vi "Set Icon.vi"(6 "Variant in":variant, 7 "Shift Pressed?":bool, 8 "error in (no error)":errorcluster, 10 "QD Combo Box Ref":refnum<vi>, 11 "QD Launch VI Ref":refnum<vi>) -> (0 "error out":errorcluster, 4 "Variant out":variant)   [LabVIEW 2017]
doc: "Replaces active VI Icon. New icon, by default, has a frame with black header and text with active VI name. Enter <b>-?</b> to display help window.\n\nDefault Shortcut - [N]"
uses:
  <vilib>/LabVIEW Icon API/API_User Layer Data.ctl
  <vilib>/Utility/miscctls.llb/LVPoint32TypeDef.ctl
  <vilib>/picture/picture.llb/imagedata.ctl
  <vilib>/LabVIEW Icon API/LabVIEW Icon API.lvlib
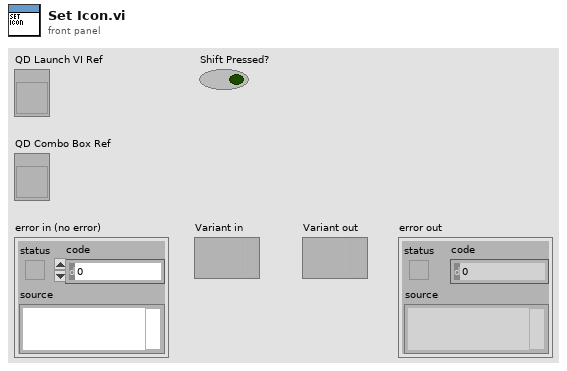
[diagram p1: front panel]
types:
  T1 = typedef "LabVIEW Icon API.lvlib/API_User Layer Data.ctl" = cluster{"Layer name":string, "Origin":T2, "Icon image data":T3}
  T2 = typedef "LVPoint32TypeDef.ctl" = cluster{"Horizontal":i32, "Vertical":i32}
  T3 = typedef "imagedata.ctl" = cluster{"image type":i32, "image depth":i32, "image":u8[], "mask":u8[], "colors":u32[], "Rectangle":cluster{"left":i16, "top":i16, "right":i16, "bottom":i16}}
  T4 = typedef "Settings.ctl" = cluster{"main text":string, "header text":string, "color":u32, "dark?":bool, "frame":T5, "format":T6, "number of lines":i32, "header?":bool, "shift":cluster{"x":i16, "y":i16}}
  T5 = typedef "Template Frame.ctl" = enum16{"none", "compact lib"}
  T6 = typedef "Text Format.ctl" = enum16{"none"}
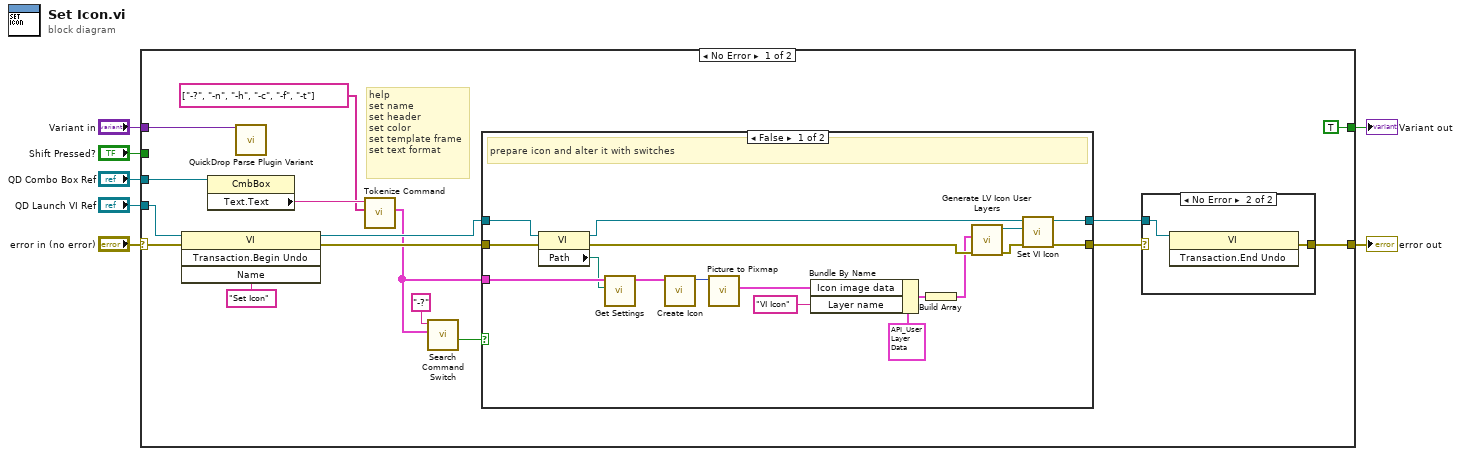
[diagram p0: block diagram]
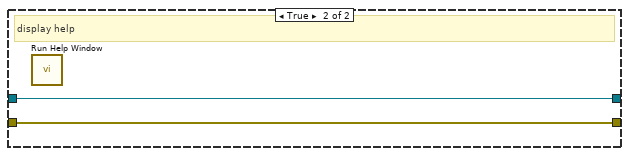
[diagram p2: hidden frame]
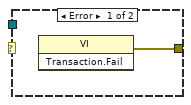
[diagram p3: hidden frame]
diagram:
  n1 = case shown="No Error" "error in (no error)" {
    selector: "error in (no error)" -> [w22 w46]
    tunnel: [w20 w46] -> w6
    tunnel: "QD Launch VI Ref" -> [w21 _]
    tunnel: "Shift Pressed?" -> [_ _]
    tunnel: "QD Combo Box Ref" -> [w18 _]
    tunnel: "Variant in" -> [w23 _]
    tunnel: [TRUE _] -> w1
    frame No Error {
      # "help\nset name\nset header\nset color\nset template frame\nset text format"
      n2 = invoke class="VI" method="Transaction.Begin Undo"(reference=w21, error in=w22, "Name"="Set Icon" ("Undo Name")) -> (reference out=w12:refnum<vi>, error out=w11:errorcluster)  [unwired: 1 in, 2 out]
      n3 = property class="CmbBox"(reference=w18) -> ("Text.Text"=w16:string)  [unwired: 1 in, 2 out]
      n4 = call <vilib>:"QuickDrop Parse Plugin Variant.vi"("QDKS Variant in"=w23) -> ()  [unwired: 12 in, 3 out]
      n5 = call "Tokenize Command.vi"("switches in"=string[] ["-?", "-n", "-h", "-c", "-f", "-t"], "command in"=w16) -> ("switches out"=w10:cluster{"switch":string, "argument":string}[])  [unwired: 7 in, 2 out]
      n6 = call "Search Command Switch.vi"("switches"=w10, "switch in"="-?" ("y")) -> ("found?"=w14:bool)  [unwired: 7 in, 2 out]
      n7 = case shown="False" w14 {
        tunnel: w10 -> [w39 _]
        tunnel: w12 -> [w38 w42]
        tunnel: w11 -> [w37 w41]
        tunnel: [w25 w42] -> w9
        tunnel: [w24 w41] -> w8
        frame False {
          # "prepare icon and alter it with switches"
          n8 = property class="VI"(reference=w38, error in=w37) -> (reference out=w29:refnum<vi>, error out=w40:errorcluster, "Path"=w36:path)
          n9 = call "Get Settings.vi"("VI path"=w36, "switches"=w39) -> ("settings"=w35:T4)  [unwired: 9 in]
          n10 = call "Create Icon.vi"("settings"=w35) -> ("new picture"=w30:picture)  [unwired: 10 in]
          n11 = call <vilib>:"Picture to Pixmap.vi"("picture"=w30) -> ("image data"=w26:T3)  [unwired: 9 in, 1 out]
          n12 = Bundle By Name(cluster=T1 {"Layer name"="", "Origin"={"Horizontal"=0, "Vertical"=0}, "Icon image data"={"image type"=0, "image depth"=0, "image"=[], "mask"=[], "colors"=[], "Rectangle"={"left"=0, "top"=0, "right"=0, "bottom"=0}}} ("User layer"), "Icon image data"=w26, "Layer name"="VI Icon") -> (w33:T1)
          n13 = Build Array(w33) -> (w32:T1[])
          n14 = call <vilib>:"Generate LV Icon User Layers.vi"("error in (no error)"=w40, "User layers"=w32) -> ("error out"=w27:errorcluster, "Icon out"=w28:refnum<class "Icon.lvclass">)  [unwired: 8 in]
          n15 = call <vilib>:"Set VI Icon.vi"("error in (no error)"=w27, "Icon"=w28, "VI Refnum in"=w29) -> ("error out"=w24:errorcluster, "VI Refnum out"=w25:refnum<vi>)  [unwired: 7 in]
        }
        frame True {
          # "display help"
          n16 = call "Run Help Window.vi"() -> ()  [unwired: 11 in, 1 out]
        }
      }
      n17 = case shown="No Error" w8 {
        tunnel: [w43 w45] -> w20
        tunnel: w9 -> [_ w44]
        frame Error {
          n18 = invoke class="VI" method="Transaction.Fail"() -> (error out=w43:errorcluster)  [unwired: 3 in, 2 out]
        }
        frame No Error {
          n19 = invoke class="VI" method="Transaction.End Undo"(reference=w44) -> (error out=w45:errorcluster)  [unwired: 2 in, 2 out]
        }
      }
    }
    frame Error {
    }
  }
  "error out" <- w6
  "Variant out" <- w1
